vi "测试报告.vi"(9 "模拟量量输入":string, 10 "数字量输出":string, 11 "数字量输入":string) -> ()   [LabVIEW 2010]
uses:
  <vilib>/Utility/NIReport.llb/NI_report.lvclass
  <vilib>/addons/_office/NI_ReportGenerationToolkit.lvlib
panel:
  out "XY图":cluster{"Y":dbl[], "Y":dbl[]}[](graph)
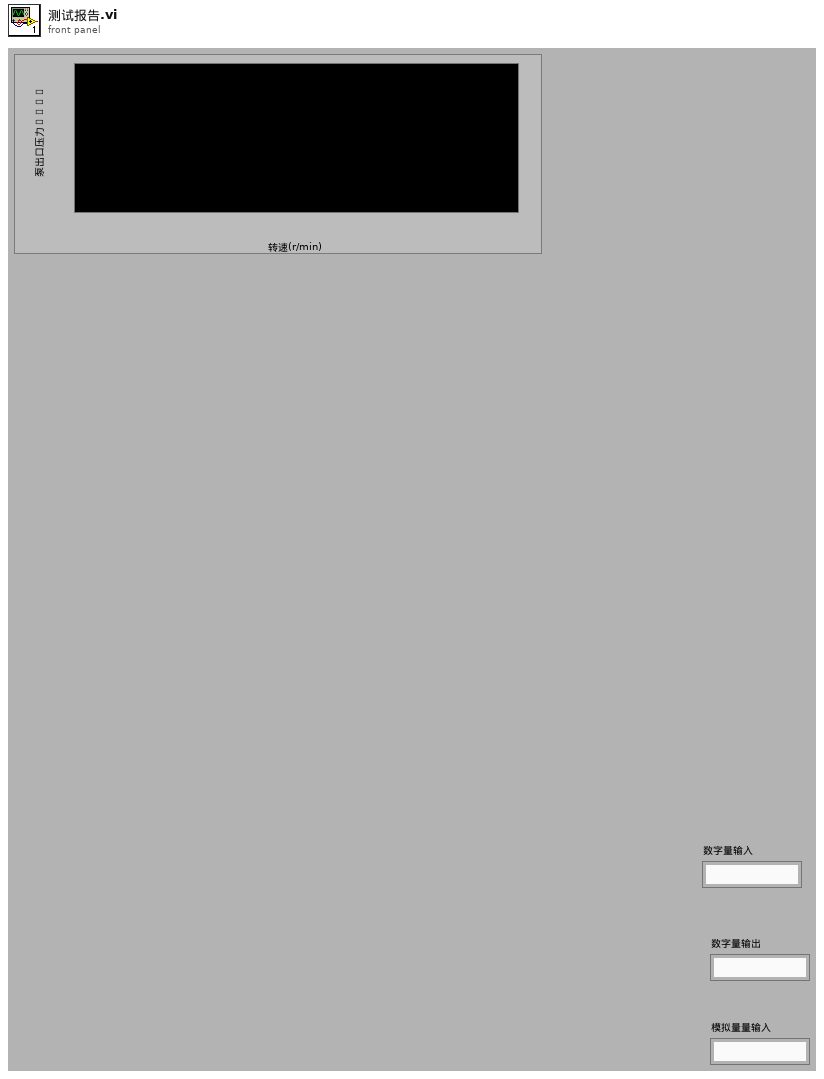
[diagram p1: front panel]
types:
  T1 = enum16{"maximized", "minimized", "normal", "no change"}
  T2 = enum16{"Standard Report", "HTML", "Word", "Excel"}
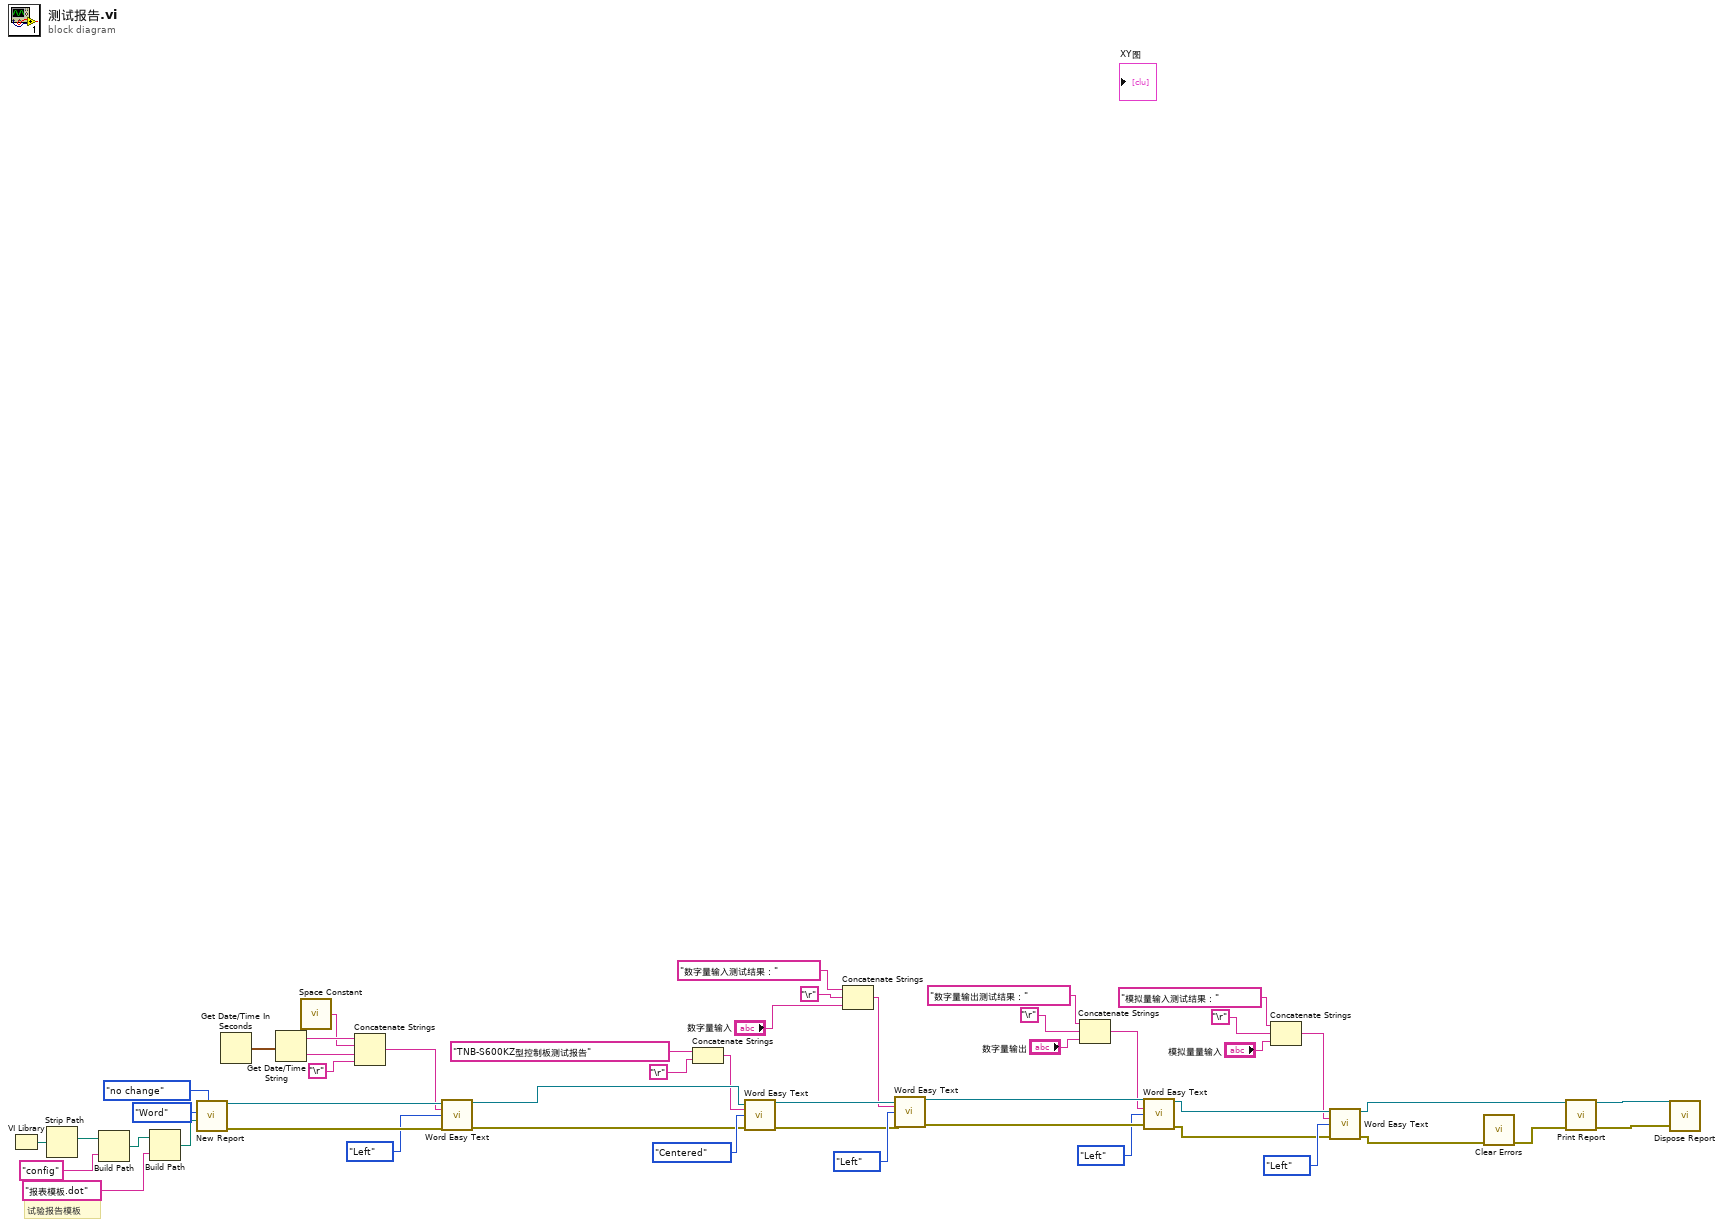
[diagram p0: block diagram]
diagram:
  # "试验报告模板"
  n1 = VI Library() -> (path=w44:path)
  n2 = Strip Path(path=w44) -> (stripped path=w47:path)  [unwired: 1 out]
  n3 = Build Path(base path=w47, name or relative path="config") -> (appended path=w45:path)
  n4 = Build Path(base path=w45, name or relative path="报表模板.dot") -> (appended path=w49:path)
  n5 = call <vilib>:"New Report.vi"("window state (normal)"=T1."no change", "report type"=T2."Word", "template (empty)"=w49) -> ("report out"=w32:refnum<class "NI_report.lvclass">, "error out"=w31:errorcluster)  [unwired: 11 in]
  n6 = Get Date/Time In Seconds() -> (seconds since 1Jan1904=w27:timestamp)
  n7 = Get Date/Time String(seconds (now)=w27) -> (date string=w26:string, time string=w25:string)  [unwired: 2 in]
  n8 = call <vilib>:"Space Constant.vi"() -> ("String"=w24:string)
  n9 = Concatenate Strings(w26, w24, w25, "\r") -> (w23:string)
  n10 = call <vilib>:"Word Easy Text.vi"("report in"=w32, "text"=w23, "alignment (left)"=enum16{"Left", "Centered", "Right", "Justify"}."Left", "error in (no error)"=w31) -> ("report out"=w30:refnum<class "NI_report.lvclass">, "error out"=w29:errorcluster)  [unwired: 9 in, 1 out]
  n11 = Concatenate Strings("TNB-S600KZ型控制板测试报告", "\r") -> (w19:string)
  n12 = call <vilib>:"Word Easy Text.vi"("report in"=w30, "text"=w19, "alignment (left)"=enum16{"Left", "Centered", "Right", "Justify"}."Centered", "error in (no error)"=w29) -> ("report out"=w34:refnum<class "NI_report.lvclass">, "error out"=w33:errorcluster)  [unwired: 9 in, 1 out]
  n13 = Concatenate Strings("数字量输入测试结果：", "\r", "数字量输入") -> (w17:string)
  n14 = call <vilib>:"Word Easy Text.vi"("report in"=w34, "text"=w17, "alignment (left)"=enum16{"Left", "Centered", "Right", "Justify"}."Left", "error in (no error)"=w33) -> ("report out"=w42:refnum<class "NI_report.lvclass">, "error out"=w43:errorcluster)  [unwired: 9 in, 1 out]
  n15 = Concatenate Strings("数字量输出测试结果：", "\r", "数字量输出") -> (w13:string)
  n16 = call <vilib>:"Word Easy Text.vi"("report in"=w42, "text"=w13, "alignment (left)"=enum16{"Left", "Centered", "Right", "Justify"}."Left", "error in (no error)"=w43) -> ("report out"=w5:refnum<class "NI_report.lvclass">, "error out"=w4:errorcluster)  [unwired: 9 in, 1 out]
  n17 = Concatenate Strings("模拟量输入测试结果：", "\r", "模拟量量输入") -> (w1:string)
  n18 = call <vilib>:"Word Easy Text.vi"("report in"=w5, "text"=w1, "alignment (left)"=enum16{"Left", "Centered", "Right", "Justify"}."Left", "error in (no error)"=w4) -> ("report out"=w3:refnum<class "NI_report.lvclass">, "error out"=w2:errorcluster)  [unwired: 9 in, 1 out]
  n19 = call <vilib>:"Clear Errors.vi"("error in (no error)"=w2) -> ("error out"=w37:errorcluster)  [unwired: 6 in]
  n20 = call-dynamic "Print Report.vi"("report in"=w3, "error in (no error)"=w37) -> ("report out"=w36:refnum<class "NI_report.lvclass">, "error out"=w35:errorcluster)  [unwired: 12 in]
  n21 = call-dynamic "Dispose Report.vi"("report in"=w36, "error in (no error)"=w35) -> ()  [unwired: 13 in, 1 out]
